vi "SA_Stop_S.vi"(5 "channelIndex":u32, 7 "systemIndex":u32, 8 "error in (no error)":errorcluster) -> (0 "error out":errorcluster)   [LabVIEW 2013]
doc: "<B>Description:</B>\nStops any ongoing movement of a positioner. Note that if a stepping movement is performed the current step is completed before the positioner is stopped. This command also stops the hold position feature of closed-loop commands, such as SA_GotoPositionAbsolute_S or even SA_FindReferenceMark_S.\nA positioner that is stopped will have a movement status of SA_STOPPED_STATUS (see SA_GetStatus_S).\n<B>Parameters:</B>\n<B>- systemIndex</B> (unsigned 32bit), input - Selects the system that the target actuator is connected to. The index is zero based.\n<B>- channelIndex</B> (unsigned 32bit), input - Selects the channel of the selected system. The index is zero based."
uses:
  MCSControl.dll
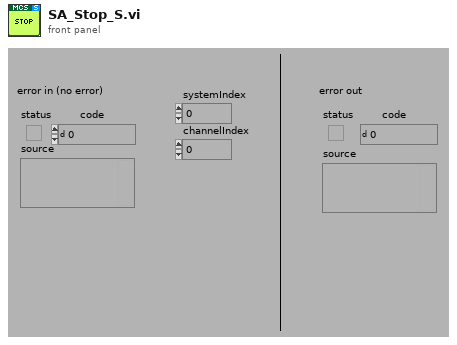
[diagram p1: front panel]
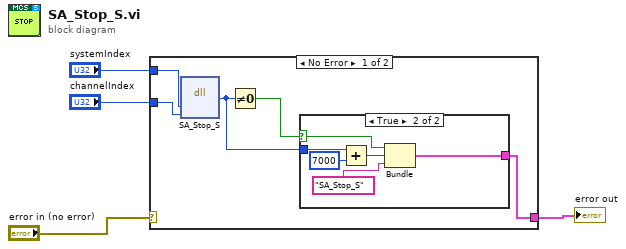
[diagram p0: block diagram]
diagram:
  n1 = case shown="No Error" "error in (no error)" {
    selector: "error in (no error)" -> [_ w16]
    tunnel: [w7 w16] -> w3
    tunnel: "systemIndex" -> [w6 _]
    tunnel: "channelIndex" -> [w5 _]
    frame No Error {
      n2 = dll-call lib="MCSControl.dll" fn="SA_Stop_S"("systemIndex"=w6, "channelIndex"=w5) -> (w8:u32)  [unwired: 5 in, 2 out]
      n3 = Not Equal To 0?(x=w8) -> (x != 0?=w9:bool)
      n4 = case shown="True" w9 {
        selector: w9 -> [_ w12]
        tunnel: w8 -> [_ w15]
        tunnel: [_ w10] -> w7
        frame False {
        }
        frame True {
          n5 = Add(x=w15, y=u32 7000) -> (x+y=w13:u32)
          n6 = Bundle(w12, w13, "source"="SA_Stop_S") -> (w10:cluster{bool, u32, "source":string})  [unwired: 1 in]
        }
      }
    }
    frame Error {
    }
  }
  "error out" <- w3
